vi "ConfigureBackChannel.vi"(8 "error in":errorcluster, 9 "backchannel remote port":u16, 10 "remote address":string, 11 "local address":string) -> (0 "error out":errorcluster, 3 "rdma session out":refnum<k21>)   [LabVIEW 2021]
uses:
  <vilib>/rdma/rdma.llb/RDMA Direction.ctl
  <vilib>/rdma/rdma.llb/RDMA Configure Buffers U8.vi
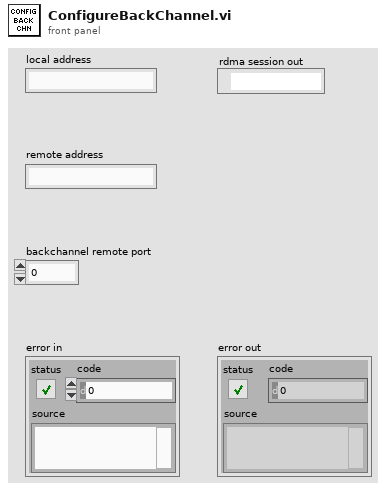
[diagram p1: front panel]
types:
  T1 = typedef "RDMA Direction.ctl" = enum16{"Send", "Receive"}
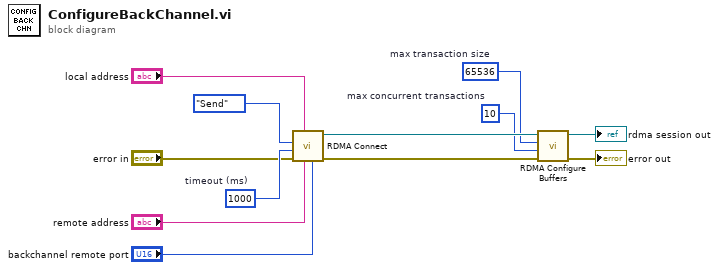
[diagram p0: block diagram]
diagram:
  w5 = u64 10  # max concurrent transactions
  w6 = u64 65536  # max transaction size
  w10 = 1000  # timeout (ms)
  n1 = call <vilib>:"RDMA Connect.vi"("remote port"="backchannel remote port", "remote address"="remote address", "local address"="local address", "error in"="error in", "timeout (ms)"=w10, "direction"=RDMA_Direction."Send") -> ("error out"=w4:errorcluster, "rdma session"=w7:refnum<k21>)  [unwired: 4 in]
  n2 = call-poly <vilib>:"RDMA Configure Buffers.vi"("error in"=w4, "max concurrent transactions"=w5, "max transaction size"=w6, "rdma session in"=w7) -> ("error out"=→"error out":errorcluster, "rdma session out"=→"rdma session out":refnum<k21>)  [unwired: 6 in]
